vi "Derivative.vi"(8 "error in (no error)":errorcluster, 11 "PID in":refnum<class "PID.lvclass">) -> (0 "error out":errorcluster, 3 "PID out":refnum<class "PID.lvclass">)   [LabVIEW 2025, in "PID.lvlib" / "PID.lvclass"]
uses:
  PID.lvclass
  PID.lvclass/PID.ctl
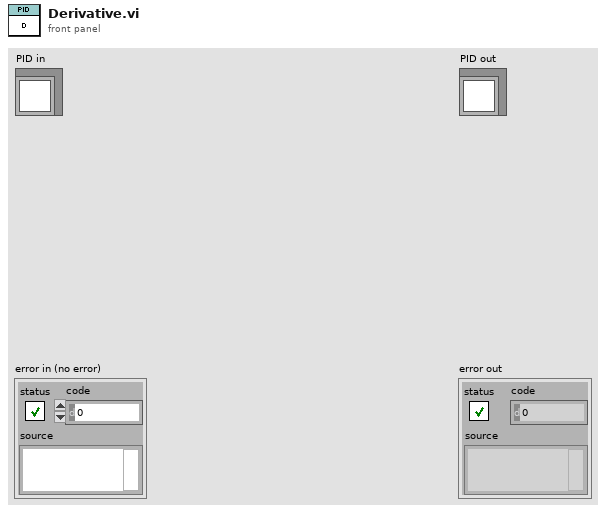
[diagram p1: front panel]
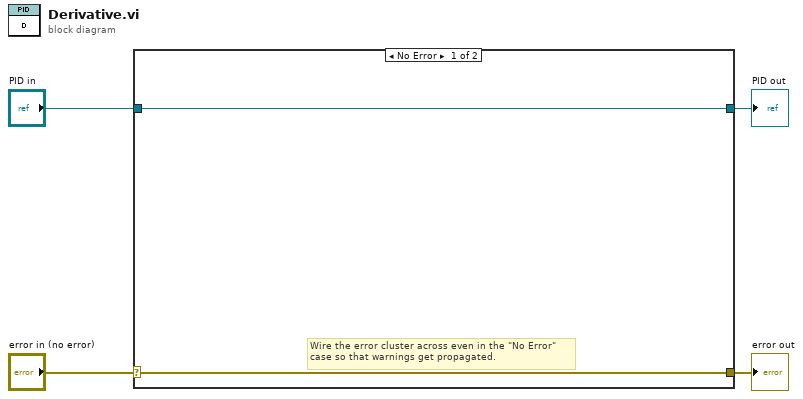
[diagram p0: block diagram]
diagram:
  n1 = case shown="No Error" "error in (no error)" {
    selector: "error in (no error)" -> [w5 w8]
    tunnel: [w5 w8] -> w3
    tunnel: [w6 w7] -> w1
    tunnel: "PID in" -> [w6 w7]
    frame No Error {
      # "Wire the error cluster across even in the \"No Error\"\ncase so that warnings get propagated."
    }
    frame Error {
    }
  }
  "error out" <- w3
  "PID out" <- w1
